vi "Izhikevich_primitive_v002.vi"(0 "UDP Network Connection in":refnum<k16>, 1 "b":dbl, 2 "a":dbl, 3 "I":dbl, 5 "c":dbl, 7 "d":dbl, 9 "v(t)":dbl, 11 "error in (no error)":errorcluster, 12 "u(t)":dbl, 13 "Numeric":dbl, 14 "Address selector":i32[](array[numeric]), 15 "Neuron ID":dbl format="%#_13g") -> (4 "UDP Network Connection out":refnum<k16>, 6 "v(t+dt)":dbl, 8 "u(t+dt)":dbl, 10 "error out":errorcluster)   [LabVIEW 2019]
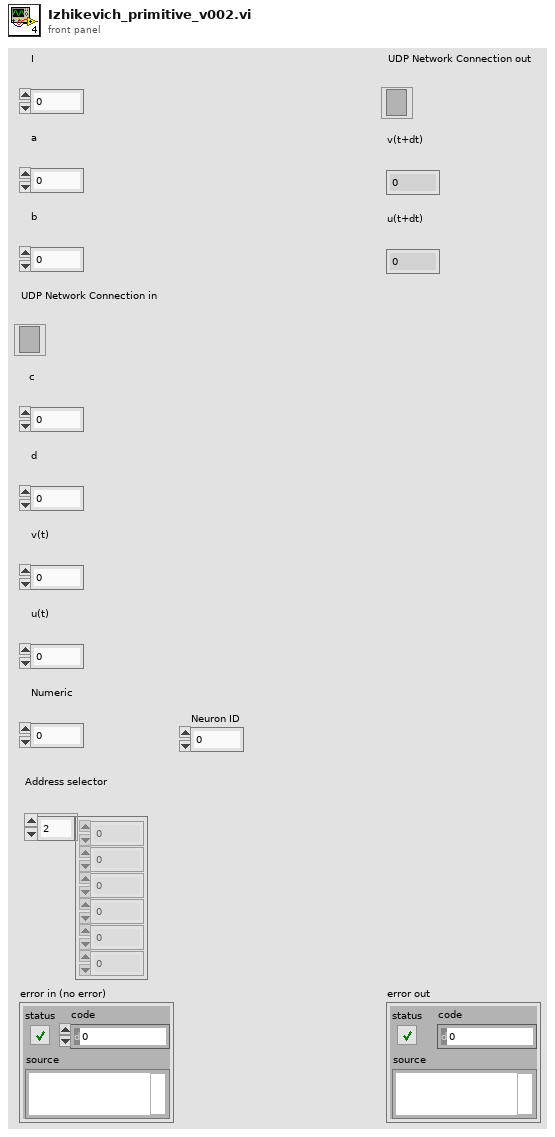
[diagram p1: front panel]
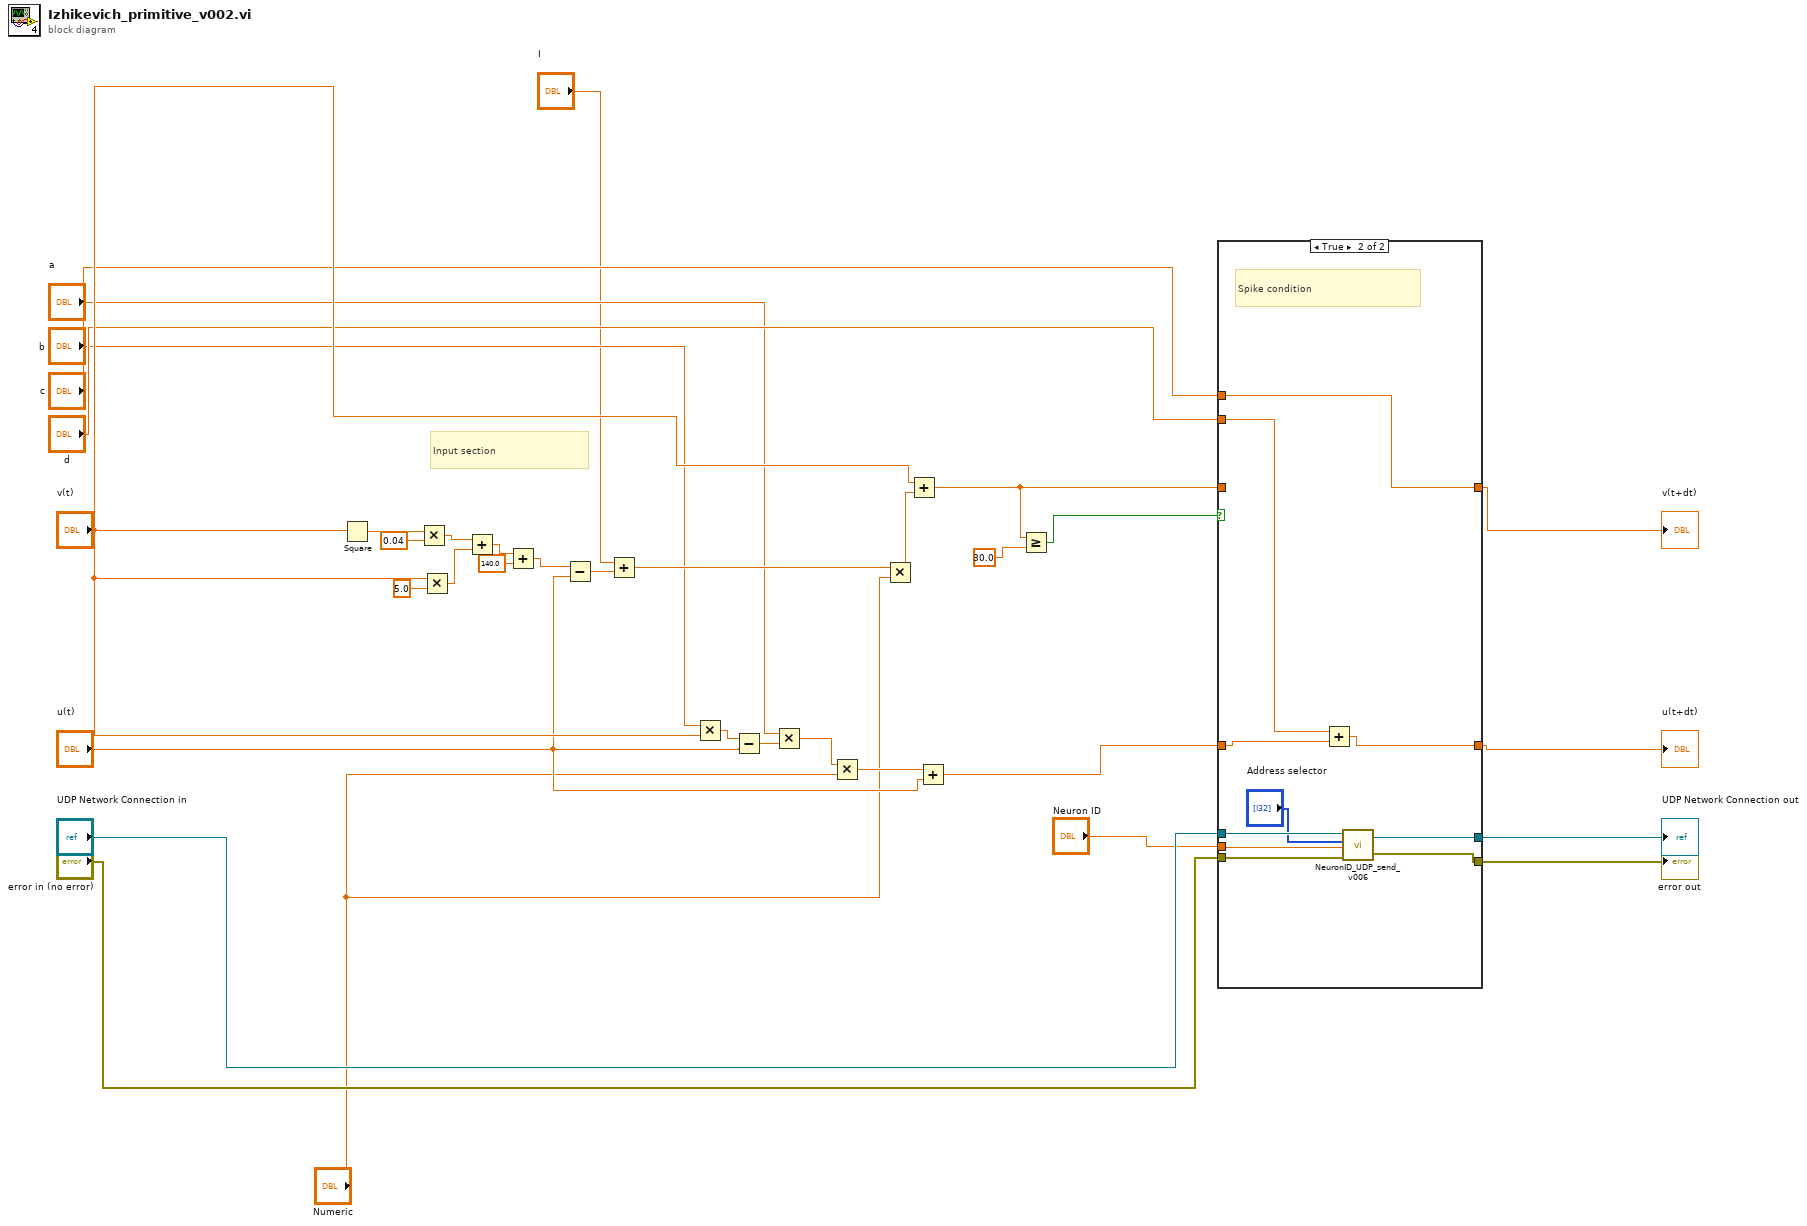
[diagram p0: block diagram]
diagram:
  # "Input section"
  n1 = Square(x="v(t)") -> (x^2=w2:dbl)
  n2 = Multiply(x=w2, y=0.04) -> (x*y=w4:dbl)
  n3 = Multiply(x="v(t)", y=5.0) -> (x*y=w6:dbl)
  n4 = Add(x=w4, y=w6) -> (x+y=w7:dbl)
  n5 = Add(x=w7, y=140.0) -> (x+y=w9:dbl)
  n6 = Subtract(x=w9, y="u(t)") -> (x-y=w10:dbl)
  n7 = Add(x="I", y=w10) -> (x+y=w17:dbl)
  n8 = Multiply(x="b", y="v(t)") -> (x*y=w13:dbl)
  n9 = Subtract(x=w13, y="u(t)") -> (x-y=w14:dbl)
  n10 = Multiply(x="a", y=w14) -> (x*y=w16:dbl)
  n11 = Multiply(x=w16, y="Numeric") -> (x*y=w20:dbl)
  n12 = Multiply(x=w17, y="Numeric") -> (x*y=w19:dbl)
  n13 = Add(x="v(t)", y=w19) -> (x+y=w29:dbl)
  n14 = Add(x=w20, y="u(t)") -> (x+y=w22:dbl)
  n15 = Greater Or Equal?(x=w29, y=30.0) -> (x >= y?=w30:bool)
  n16 = case shown="True" w30 {
    tunnel: [w38 w45] -> w21
    tunnel: w22 -> [w38 w47]
    tunnel: w29 -> [w37 _]
    tunnel: [w37 w48] -> w23
    tunnel: "c" -> [_ w48]
    tunnel: "d" -> [_ w46]
    tunnel: [w36 w42] -> w31
    tunnel: "error in (no error)" -> [w36 w43]
    tunnel: "UDP Network Connection in" -> [w35 w44]
    tunnel: [w35 w39] -> w33
    tunnel: "Neuron ID" -> [_ w41]
    frame False {
      # "No spike condition"
    }
    frame True {
      # "Spike condition"
      n17 = Add(x=w46, y=w47) -> (x+y=w45:dbl)
      n18 = call "NeuronID_UDP_send_v006.vi"("error in (no error)"=w43, "Neuron ID"=w41, "Address selector"="Address selector", "UDP Network Connection in"=w44) -> ("error out"=w42:errorcluster, "UDP Network Connection out"=w39:refnum<k16>)
    }
  }
  "UDP Network Connection out" <- w33
  "error out" <- w31
  "v(t+dt)" <- w23
  "u(t+dt)" <- w21
